vi "Run.vi"(9 "Team In":refnum<class "Team.lvclass">, 11 "MySquare in":refnum<class "MySquare.lvclass">) -> (1 "Team":refnum<class "Team.lvclass">, 2 "Run Result":T1, 3 "MySquare out":refnum<class "MySquare.lvclass">)   [LabVIEW 2020, in "DNattTeam.lvlib" / "MySquare.lvclass"]
doc: "This VI is called on every active square each turn of the game for the square to decide what action to take."
uses:
  MySquare.lvclass
  C:/Apps/GIE/Instructions Test/SquareBattle/Square/Square.lvclass
  SquareBattle/Run Result.ctl
  SquareBattle/Square/Square.lvclass
  SquareBattle/Action.ctl
  SquareBattle/Direction.ctl
  SquareBattle/Team/Team.lvclass
  MyTeam/MyTeam.lvclass
  C:/Apps/GIE/Instructions Test/SquareBattle/Team/Team.lvclass
  SquareBattle/Square/Square.lvclass/Square.ctl
  <vilib>/numeric/Random Number (Range) U64.vi
  <vilib>/numeric/sub_Random U32.vi
  SquareBattle/SquareBattle.lvlib
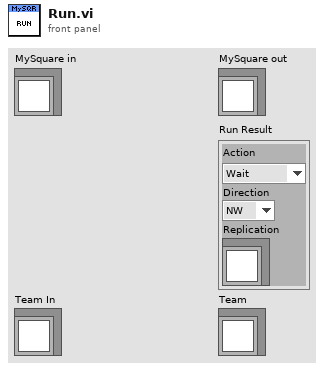
[diagram p1: front panel]
types:
  T1 = typedef "SquareBattle.lvlib/Run Result.ctl" = cluster{"Action":T2, "Direction":T3, "Replication":refnum<class "Square.lvclass">}
  T2 = typedef "SquareBattle.lvlib/Action.ctl" = enum16{"Wait", "Move", "Attack", "Replicate"}
  T3 = typedef "SquareBattle.lvlib/Direction.ctl" = enum16{"NW", "N", "NE", "E", "SE", "S", "SW", "W"}
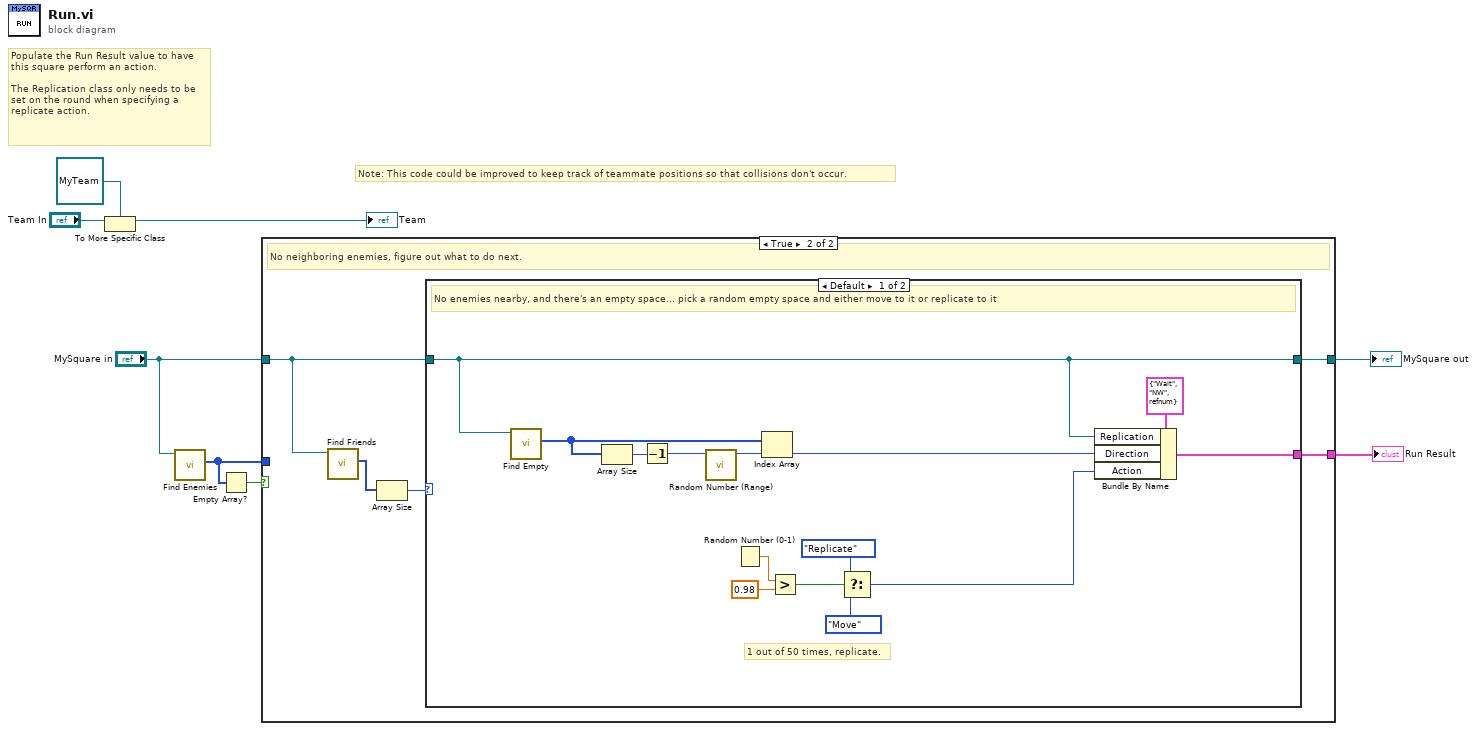
[diagram p0: block diagram]
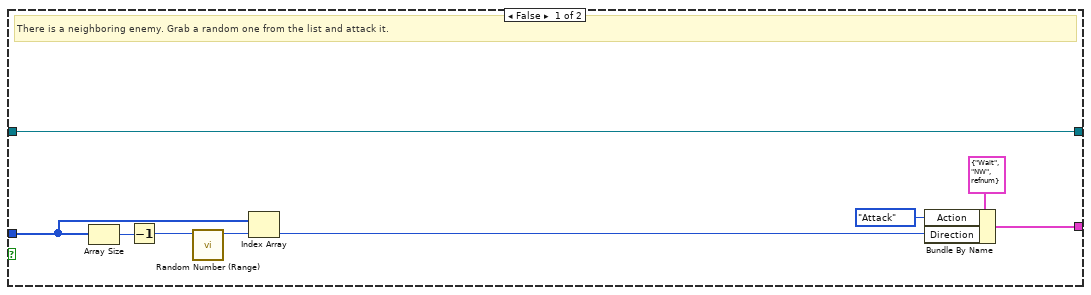
[diagram p2: hidden frame]
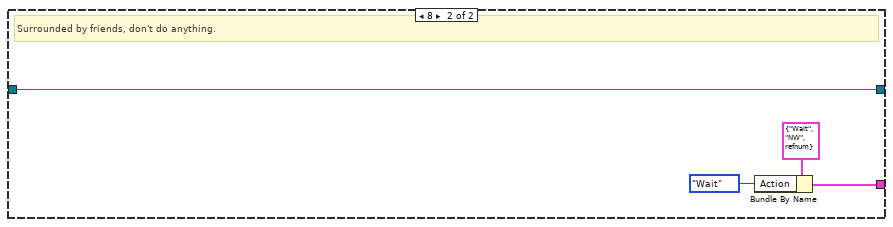
[diagram p3: hidden frame]
diagram:
  # "Note: This code could be improved to keep track of teammate positions so that collisions don't occur."
  # "Populate the Run Result value to have this square perform an action.\n\nThe Replication class only needs to be set on the round when specifying a replicate action."
  n1 = To More Specific Class(target class=refnum<class "MyTeam.lvclass"> refnum ("SquareTeam.lvlib:MyTeam.lvclass"), reference="Team In") -> (specific class reference=→"Team":refnum<class "MyTeam.lvclass">)  [unwired: 1 in, 1 out]
  n2 = call "Find Enemies.vi"("Square"="MySquare in") -> ("Enemy Directions"=w4:T3[])  [unwired: 10 in]
  n3 = Empty Array?(array=w4) -> (empty?=w5:bool)
  n4 = case shown="True" w5 {
    tunnel: "MySquare in" -> [w9 w19]
    tunnel: w4 -> [w14 _]
    tunnel: [w12 w18] -> w3
    tunnel: [w9 w20] -> w2
    frame False {
      # "There is a neighboring enemy. Grab a random one from the list and attack it."
      n5 = Array Size(array=w14) -> (size(s)=w17:i32)
      n6 = Decrement(x=w17) -> (x-1=w16:i32)
      n7 = call-poly <vilib>:"Random Number (Range).vi"("upper bound (100)"=w16) -> ("number"=w15:u64)  [unwired: 10 in]
      n8 = Index Array(array=w14, index=w15) -> (element=w11:T3)
      n9 = Bundle By Name(cluster=T1 {"Action"=enum."Wait", "Direction"=enum."NW", "Replication"=refnum} ("Run Result"), "Action"=Action."Attack", "Direction"=w11) -> (w12:T1)
    }
    frame True {
      # "No neighboring enemies, figure out what to do next."
      n10 = call "Find Friends.vi"("Square in"=w19) -> ("Friend Directions"=w22:T3[])  [unwired: 10 in]
      n11 = Array Size(array=w22) -> (size(s)=w21:i32)
      n12 = case shown="Default" w21 {
        tunnel: [w23 w40] -> w20
        tunnel: w19 -> [w23 w40]
        tunnel: [w26 w37] -> w18
        frame Default {
          # "1 out of 50 times, replicate."
          # "No enemies nearby, and there's an empty space... pick a random empty space and either move to it or replicate to it"
          n13 = call "Find Empty.vi"("Square"=w23) -> ("Empty Directions"=w33:T3[])  [unwired: 10 in]
          n14 = Array Size(array=w33) -> (size(s)=w36:i32)
          n15 = Decrement(x=w36) -> (x-1=w35:i32)
          n16 = call-poly <vilib>:"Random Number (Range).vi"("upper bound (100)"=w35) -> ("number"=w34:u64)  [unwired: 10 in]
          n17 = Random Number (0-1)() -> (number: 0 to 1=w32:dbl)
          n18 = Index Array(array=w33, index=w34) -> (element=w24:T3)
          n19 = Greater?(x=w32, y=0.98) -> (0:w29:bool)
          n20 = Select(t=Action."Replicate" ("Action"), s=w29, f=Action."Move" ("Action")) -> (s? t:f=w25:T2)
          n21 = Bundle By Name(cluster=T1 {"Action"=enum."Wait", "Direction"=enum."NW", "Replication"=refnum} ("Run Result"), "Replication"=w23, "Direction"=w24, "Action"=w25) -> (w26:T1)
        }
        frame 8 {
          # "Surrounded by friends, don't do anything."
          n22 = Bundle By Name(cluster=T1 {"Action"=enum."Wait", "Direction"=enum."NW", "Replication"=refnum} ("Run Result"), "Action"=Action."Wait") -> (w37:T1)
        }
      }
    }
  }
  "MySquare out" <- w2
  "Run Result" <- w3
